vi "Rucker And Kolls 683A.vi"() -> ()   [LabVIEW 2015]
uses:
  <vilib>/Utility/file.llb/Read Delimited Spreadsheet (string).vi
  <vilib>/Utility/file.llb/Write Delimited Spreadsheet (string).vi
panel:
  out "CVolt":dbl
  in  "Output Filepath":path
  out "Readings":string[][](table)
  in  "Max (V)":dbl
  in  "Min (V)":dbl
  in  "Step (V)":dbl
  out "Keithley Name":string
  out "HP Name":string
  out "RK Name":string
  out "List_Test":i32(listbox)
  in  "Log":string
  out "Running":bool
  in  "Start / Stop":bool
  in  "Down":bool
  in  "Right":bool
  in  "Left":bool
  in  "Up":bool
  out "Table":string[][](table)
  in  "Boxes CSV File":path
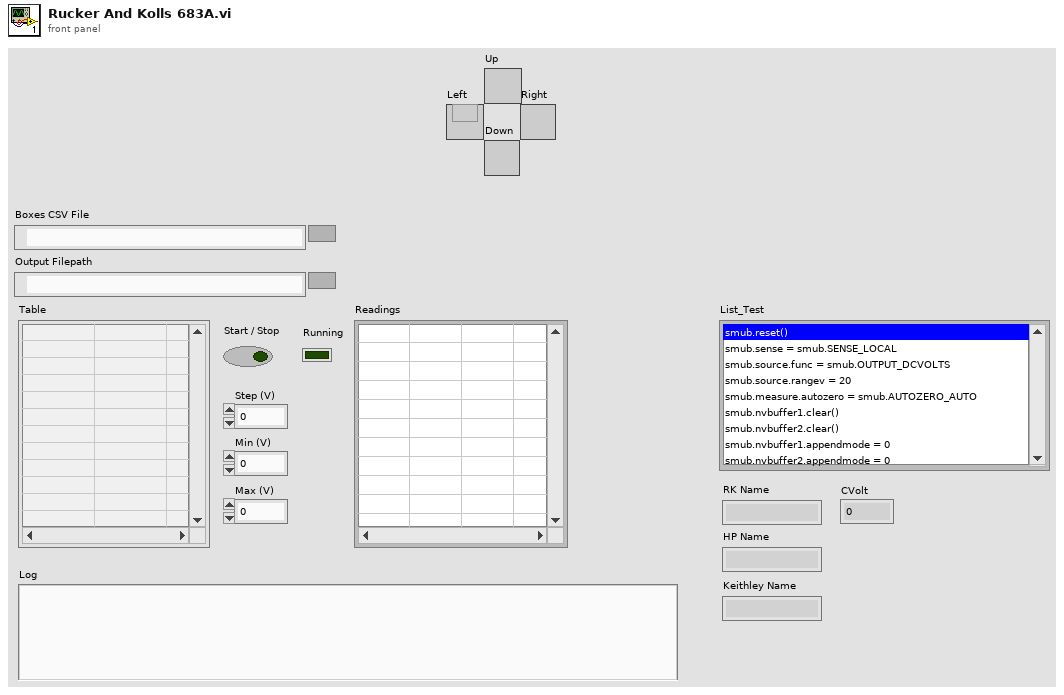
[diagram p1: front panel]
types:
  T1 = cluster{"output string":string, "result string":string, "result string":string}
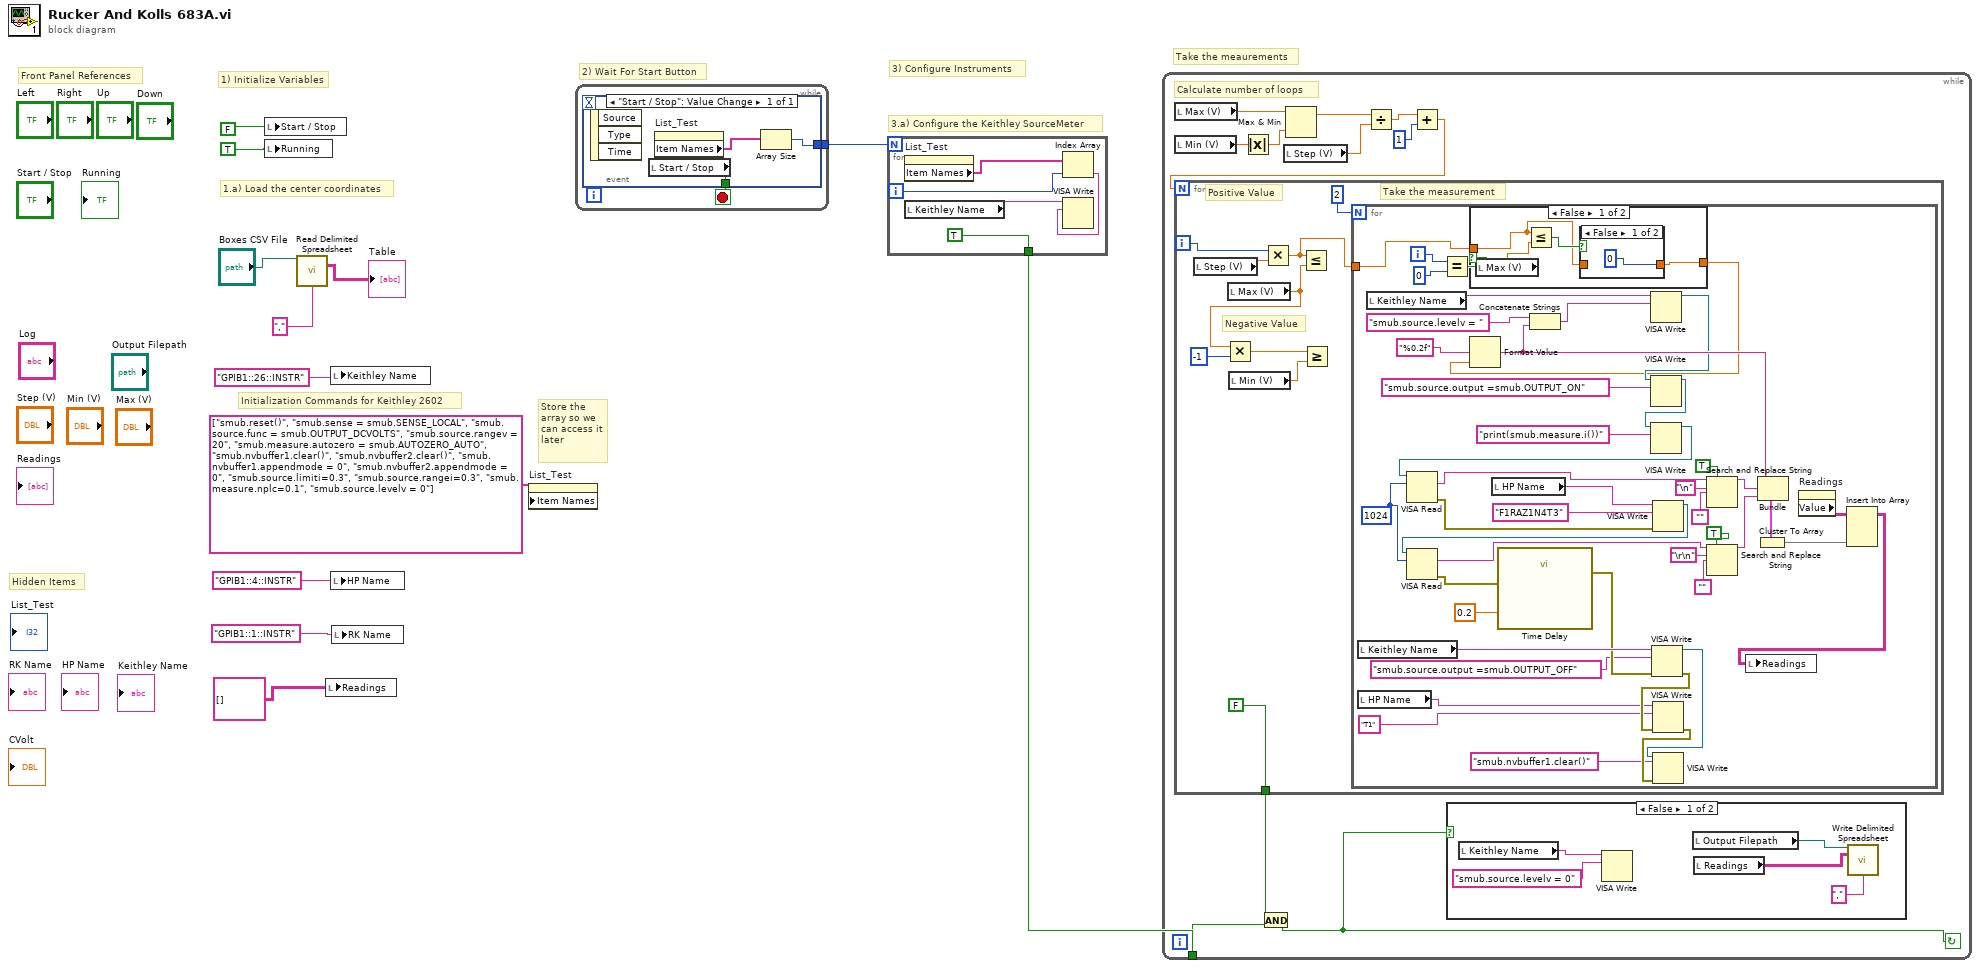
[diagram p0: block diagram]
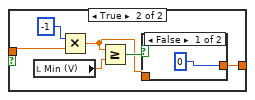
[diagram p4: hidden frame]
diagram:
  # "Take the meaurements"
  # "Store the array so we can access it later"
  # "1.a) Load the center coordinates"
  # "3.a) Configure the Keithley SourceMeter"
  # "Hidden Items"
  # "3) Configure Instruments"
  # "2) Wait For Start Button"
  # "Initialization Commands for Keithley 2602"
  # "1) Initialize Variables"
  # "Front Panel References"
  n1 = local write "Start / Stop"(FALSE) -> ()
  n2 = local write "Running"(TRUE) -> ()
  n3 = call-poly <vilib>:"Read Delimited Spreadsheet.vi"("file path (dialog if empty)"="Boxes CSV File", "delimiter (\\t)"="," ("String")) -> ("all rows"=→"Table":string[][])  [unwired: 8 in, 5 out]
  n4 = local write "Readings"(string[][] []) -> ()
  n5 = local write "Keithley Name"("GPIB1::26::INSTR") -> ()
  n6 = local write "HP Name"("GPIB1::4::INSTR") -> ()
  n7 = local write "RK Name"("GPIB1::1::INSTR") -> ()
  n8 = property on="List_Test" class="LstBox (strict)"("Item Names"=string[] ["smub.reset()", "smub.sense = smub.SENSE_LOCAL", "smub.source.func = smub.OUTPUT_DCVOLTS", "smub.source.rangev = 20", "smub.measure.autozero = smub.AUTOZERO_AUTO", "smub.nvbuffer1.clear()", "smub.nvbuffer2.clear()", "smub.nvbuffer1.appendmode = 0", "smub.nvbuffer2.appendmode = 0", "smub.source.limiti=0.3", "smub.source.rangei=0.3", "smub.measure.nplc=0.1", "smub.source.levelv = 0"]) -> ()  [unwired: 2 in, 2 out]
  n9 = while {
    tunnel: [w13] -> w6
    stop <- w14 stop-if-true
    n10 = event shown="[0] \"Start / Stop\": Value Change" {
      selector: _ -> [_]
      dyn-events: _ -> [_]
      timeout: _ -> [_]
      tunnel: [w16] -> w14
      tunnel: [w17] -> w13
      event "Start / Stop": Value Change {
        n11 = event-data() -> ()  [unwired: 1 in, 3 out]
        n12 = local read "Start / Stop"() -> (w16:bool)
        n13 = property on="List_Test" class="LstBox (strict)"() -> ("Item Names"=w15:string[])  [unwired: 2 in, 2 out]
        n14 = Array Size(array=w15) -> (size(s)=w17:i32)
      }
    }
  }
  n15 = for {
    N: w6 -> [_]
    tunnel: [TRUE] -> w2
    i -> [w19]
    n16 = property on="List_Test" class="LstBox (strict)"() -> ("Item Names"=w20:string[])  [unwired: 2 in, 2 out]
    n17 = local read "Keithley Name"() -> (w22:string)
    n18 = Index Array(array=w20, index=w19) -> (element=w21:string)
    n19 = VISA Write(VISA resource name=w22, write buffer=w21) -> ()  [unwired: 1 in, 3 out]
  }
  n20 = while {
    tunnel: w2 -> [w27]
    stop <- w23 continue-if-true
    # "Calculate number of loops"
    n21 = local read "Max (V)"() -> (w31:dbl)
    n22 = local read "Min (V)"() -> (w33:dbl)
    n23 = Absolute Value(x=w33) -> (abs(x)=w32:dbl)
    n24 = local read "Step (V)"() -> (w29:dbl)
    n25 = Max & Min(x=w31, y=w32) -> (max(x,y)=w30:dbl)  [unwired: 1 out]
    n26 = Divide(x=w30, y=w29) -> (x/y=w26:dbl)
    n27 = Add(x=w26, y=1) -> (x+y=w24:dbl)
    n28 = for {
      N: w24 -> [_]
      tunnel: [FALSE] -> w28
      i -> [w41]
      # "Take the measurement"
      # "Negative Value"
      # "Positive Value"
      n29 = local read "Step (V)"() -> (w47:dbl)
      n30 = local read "Max (V)"() -> (w46:dbl)
      n31 = Multiply(x=w46, y=-1) -> (x*y=w44:dbl)
      n32 = local read "Min (V)"() -> (w43:dbl)
      n33 = Multiply(x=w41, y=w47) -> (x*y=w42:dbl)
      n34 = Less Or Equal?(x=w42, y=w46) -> ()  [unwired: 1 out]
      n35 = Greater Or Equal?(x=w44, y=w43) -> ()  [unwired: 1 out]
      n36 = for {
        N: 2 -> [_]
        tunnel: w42 -> [w59]
        i -> [w62]
        w81 = 1024
        n37 = local read "Keithley Name"() -> (w79:string)
        n38 = local read "HP Name"() -> (w74:string)
        n39 = local read "Keithley Name"() -> (w88:string)
        n40 = Equal?(x=w62, y=0) -> (x = y?=w60:bool)
        n41 = case shown="False" w60 {
          tunnel: w59 -> [w94 w102]
          tunnel: [w93 w99] -> w58
          frame False {
            n42 = local read "Max (V)"() -> (w96:dbl)
            n43 = Less Or Equal?(x=w94, y=w96) -> (x <= y?=w95:bool)
            n44 = case shown="False" w95 {
              tunnel: w94 -> [_ w98]
              tunnel: [0 w98] -> w93
              frame False {
              }
              frame True {
              }
            }
          }
          frame True {
            n45 = local read "Min (V)"() -> (w101:dbl)
            n46 = Multiply(x=-1, y=w102) -> (x*y=w100:dbl)
            n47 = Greater Or Equal?(x=w100, y=w101) -> (x >= y?=w104:bool)
            n48 = case shown="False" w104 {
              tunnel: w100 -> [_ w106]
              tunnel: [0 w106] -> w99
              frame False {
              }
              frame True {
              }
            }
          }
        }
        n49 = Format Value(format string="%0.2f", value (0)=w58) -> (output string=w64:string)  [unwired: 1 in]
        n50 = local read "HP Name"() -> (w84:string)
        n51 = Concatenate Strings("smub.source.levelv = ", w64) -> (w92:string)
        n52 = VISA Write(VISA resource name=w88, write buffer=w92) -> (VISA resource name out=w63:refnum<visa-resource-name>)  [unwired: 1 in, 2 out]
        n53 = VISA Write(VISA resource name=w63, write buffer="smub.source.output =smub.OUTPUT_ON") -> (VISA resource name out=w87:refnum<visa-resource-name>)  [unwired: 1 in, 2 out]
        n54 = VISA Write(VISA resource name=w87, write buffer="print(smub.measure.i())") -> (VISA resource name out=w86:refnum<visa-resource-name>)  [unwired: 1 in, 2 out]
        n55 = VISA Read(VISA resource name=w86, byte count=w81) -> (read buffer=w57:string, error out=w85:errorcluster)  [unwired: 1 in, 2 out]
        n56 = VISA Write(VISA resource name=w84, write buffer="F1RAZ1N4T3", error in (no error)=w85) -> (VISA resource name out=w82:refnum<visa-resource-name>)  [unwired: 2 out]
        n57 = VISA Read(VISA resource name=w82, byte count=w81) -> (read buffer=w52:string, error out=w80:errorcluster)  [unwired: 1 in, 2 out]
        n58 = call "Time Delay"("error in (no error)"=w80, "Delay Time (s)"=0.2) -> ("error out"=w78:errorcluster)  [unwired: 9 in]
        n59 = VISA Write(VISA resource name=w79, write buffer="smub.source.output =smub.OUTPUT_OFF", error in (no error)=w78) -> (VISA resource name out=w72:refnum<visa-resource-name>, error out=w75:errorcluster)  [unwired: 1 out]
        n60 = VISA Write(VISA resource name=w74, write buffer="T1", error in (no error)=w75) -> (error out=w71:errorcluster)  [unwired: 2 out]
        n61 = VISA Write(VISA resource name=w72, write buffer="smub.nvbuffer1.clear()", error in (no error)=w71) -> ()  [unwired: 3 out]
        n62 = Search and Replace String(replace all?=TRUE, input string=w57, search string="\n", replace string="") -> (result string=w56:string)  [unwired: 4 in, 3 out]
        n63 = Search and Replace String(replace all?=TRUE, input string=w52, search string="\r\n", replace string="") -> (result string=w49:string)  [unwired: 4 in, 3 out]
        n64 = Bundle("output string"=w64, "result string"=w56, "result string"=w49) -> (w68:T1)  [unwired: 1 in]
        n65 = Cluster To Array(cluster=w68) -> (array=w67:string[])
        n66 = property on="Readings" class="Tbl (strict)"() -> ("Value"=w69:string[][])  [unwired: 2 in, 2 out]
        n67 = Insert Into Array "Insert Into Array"(array=w69, new element=w67) -> (w66:string[][])  [unwired: 2 in]
        n68 = local write "Readings"(w66) -> ()
      }
    }
    n69 = And(x=w28, y=w27) -> (x .and. y?=w23:bool)
    n70 = case shown="False" w23 {
      frame False {
        n71 = local read "Keithley Name"() -> (w35:string)
        n72 = VISA Write(VISA resource name=w35, write buffer="smub.source.levelv = 0") -> ()  [unwired: 1 in, 3 out]
        n73 = local read "Output Filepath"() -> (w37:path)
        n74 = local read "Readings"() -> (w36:string[][])
        n75 = call-poly <vilib>:"Write Delimited Spreadsheet.vi"("file path (dialog if empty)"=w37, "2D data"=w36, "delimiter (\\t)"=",") -> ()  [unwired: 11 in, 2 out]
      }
      frame True {
      }
    }
  }
